vi "PRIVATE.panel.vi"() -> ()   [LabVIEW 2014]
doc: "example GUI for a class inherited from the DeviceBaseGUI\n\nauthor: Dietrich Beck, GSI\nlicense: GPL"
uses:
  CSCore/CSSystem/CoreLib/CoreLib.lvlib
  CSCore/CSObj/CSObj.lvlib
  CSlibraries/UtilityLib/UtilityLib.lvlib
  CSCore/CSApplicationBaseClasses/DeviceBase/DeviceBase.lvlib
  CSCore/CSSystem/CoreLib/CoreLib.short 2 byte array.vi
  CSCore/CSSystem/CoreLib/CoreLib.string 2 byte array.vi
  CSlibraries/UtilityLib/UtilityLib.valueStatus.ctl
  lib.lib/DimLVEvent/DimIndicators/DimIndicators.numericType.ctl
  lib.lib/DimLVEvent/DimIndicators/DimIndicators.anyType.ctl
panel:
  in  "Set":bool
  out "Busy":bool
  out "ErrorString":string
  out "deviceIDString":string
  in  "tab":enum32{"standard", "advanced"}(tab)
  in  "function":u16(ring) items=["choose function", "Initialize", "Close", "Configure", "Reset", "IDQuery"]
  in  "advancedGUI":bool
  out "loop counter":i32
  out "error out":errorcluster
  in  "error in (no error)":errorcluster
  in  "object ref":refnum<vi>
  in  "state":T1 caption="dic_service_numeric"
  in  "deviceID":T2 caption="dic_service_anyType"
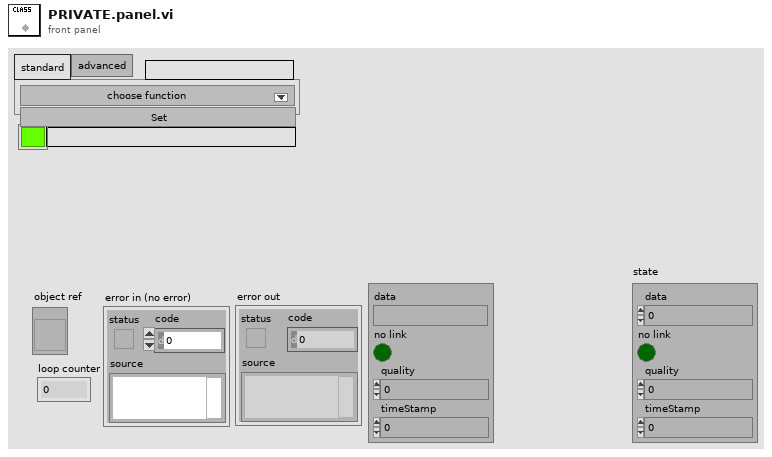
[diagram p1: front panel]
types:
  T1 = typedef "DimIndicators.lvlib/DimIndicators.numericType.ctl" = cluster{"data":dbl, "no link":bool, "quality":i32, "timeStamp":dbl}
  T2 = typedef "DimIndicators.lvlib/DimIndicators.anyType.ctl" = cluster{"data":string, "no link":bool, "quality":i32, "timeStamp":dbl}
  T3 = typedef "UtilityLib.lvlib/UtilityLib.valueStatus.ctl" = enum16{"no info available", "stand by/off", "on", "warning", "alarm/malfunction", "not implemented", "user action required", "important information", "system default", "control default", "indicator default", "button default"}
  T4 = typedef "DeviceBaseGUI.lvlib/DeviceBaseGUI.i attribute.ctl" = cluster{"GOGFrontPanel.i attribute":T5}
  T5 = typedef "GOGFrontPanel.lvlib/GOGFrontPanel.i attribute.ctl" = cluster{"GOGObject":string, "Object":string, "Method":string, "Descriptor":T6, "Input Descriptor":string, "Output Descriptor":string, "inputNames":string[], "outputNames":string[], "Values":cluster{"descriptor":string, "value":string}[]}
  T6 = typedef "BaseProcess.lvlib/BaseProcess.descriptor string definition.ctl" = string
  T7 = typedef "CoreDefs.rawDataType.ctl" = i8[]
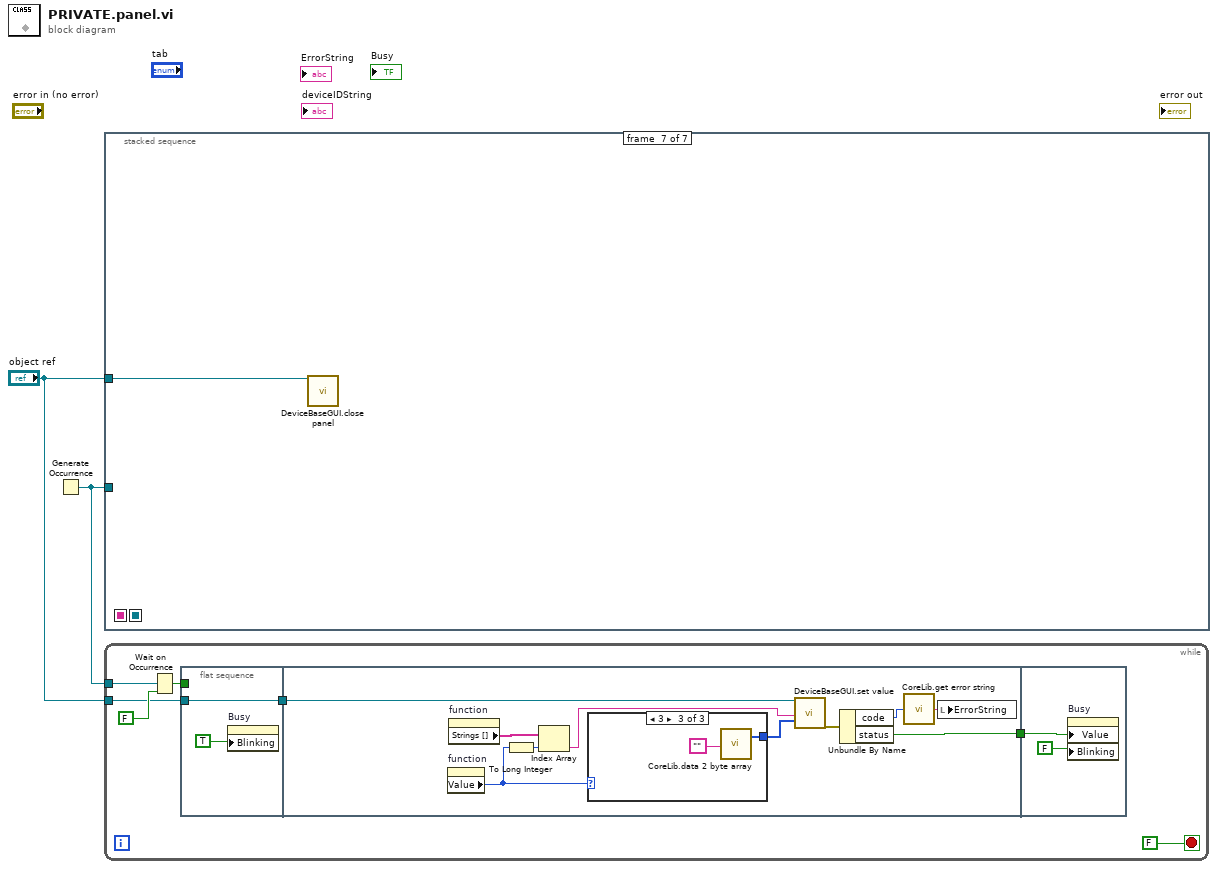
[diagram p0: block diagram]
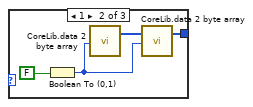
[diagram p3: hidden frame]
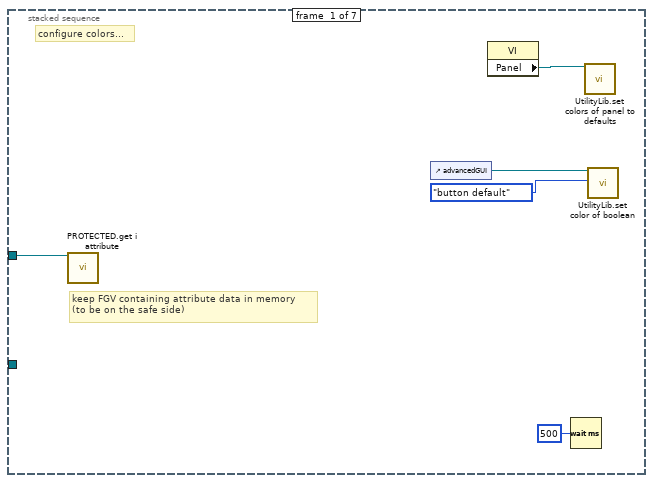
[diagram p4: hidden frame]
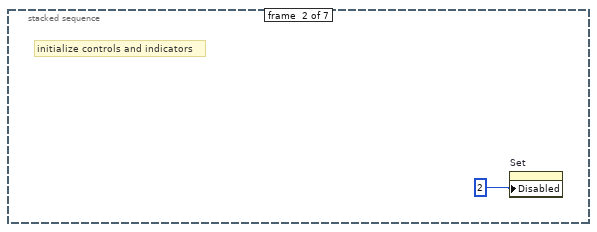
[diagram p5: hidden frame]
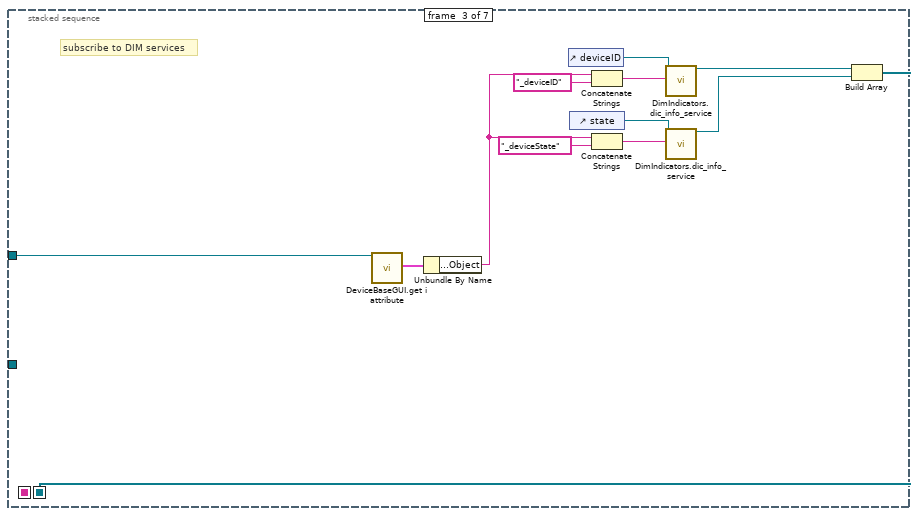
[diagram p6: hidden frame]
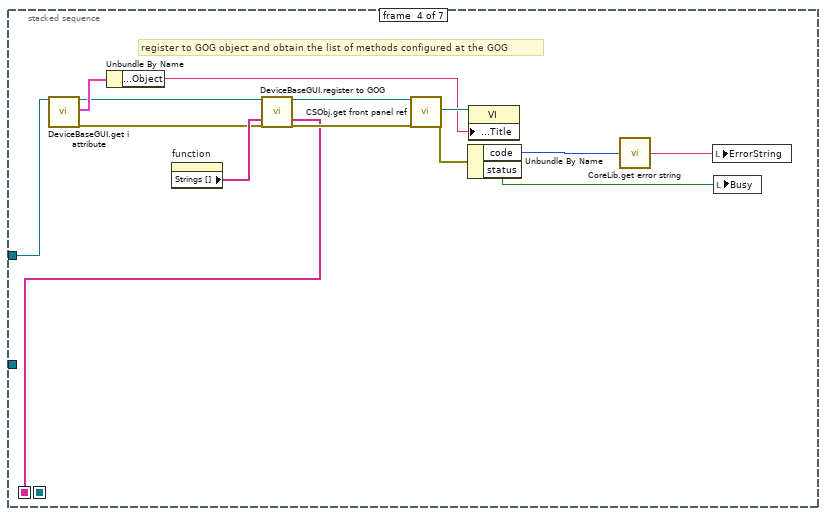
[diagram p7: hidden frame]
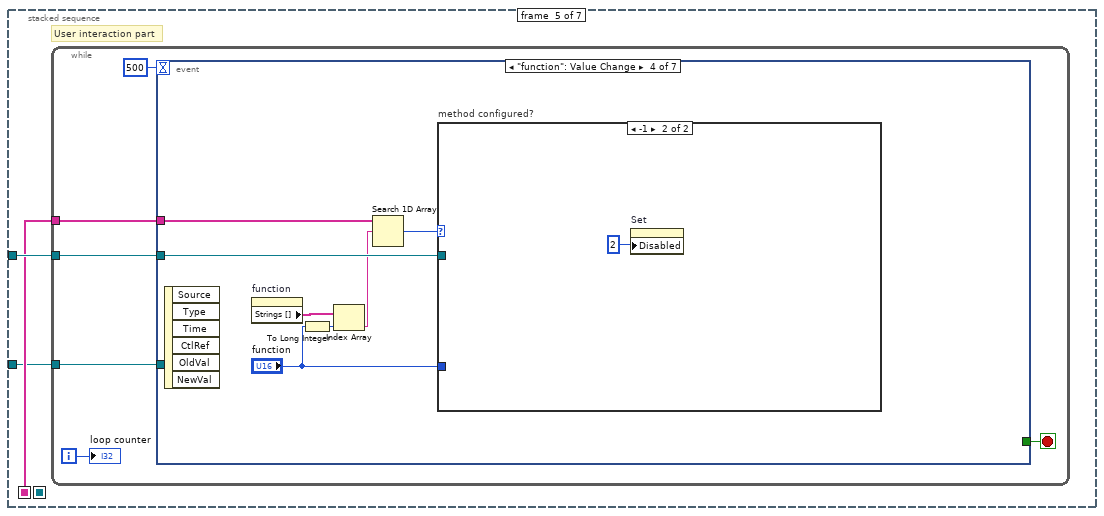
[diagram p8: hidden frame]
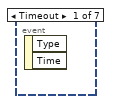
[diagram p9: hidden frame]
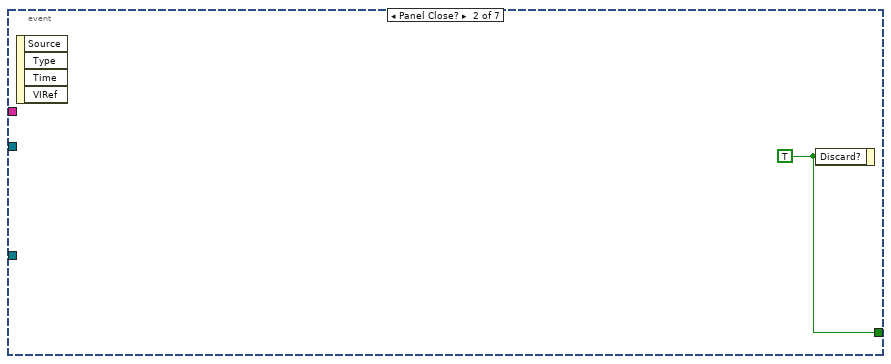
[diagram p10: hidden frame]
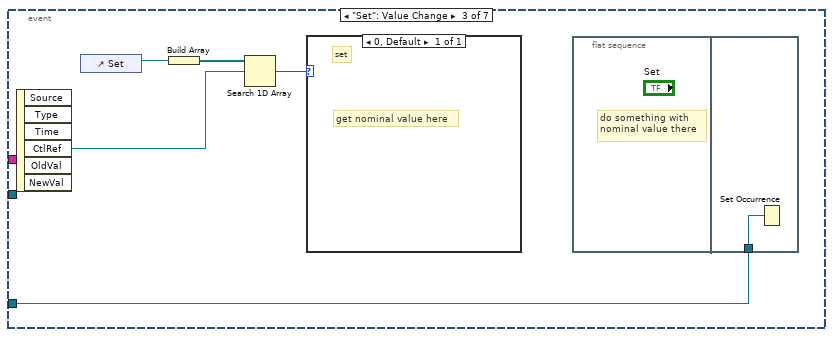
[diagram p11: hidden frame]
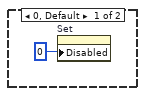
[diagram p12: hidden frame]
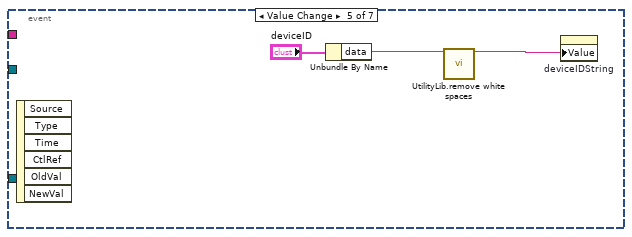
[diagram p13: hidden frame]
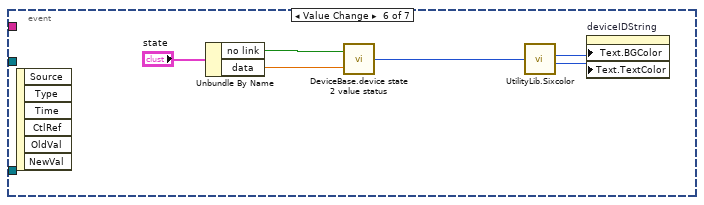
[diagram p14: hidden frame]
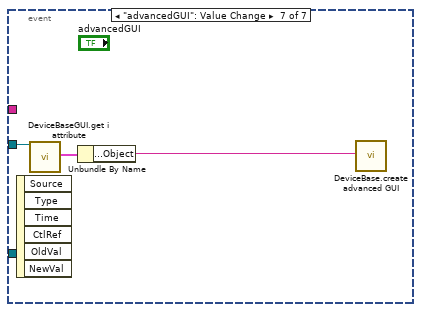
[diagram p15: hidden frame]
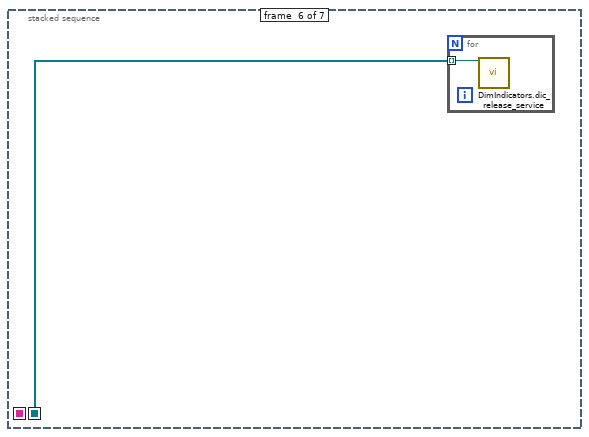
[diagram p16: hidden frame]
diagram:
  n1 = Generate Occurrence() -> (w1:refnum<k4>)
  n2 = stacked-sequence {
    seq-local: [_ _ _ w25 _ _ _] -> [_ _ _ _ w36 _ _]
    seq-local: [_ _ w9 _ _ _ _] -> [_ _ _ _ _ w72 _]
    tunnel: "object ref" -> [w3 _ w20 w34 w37 _ w74]
    tunnel: w1 -> [_ _ _ _ w35 _ _]
    frame #0 {
      # "keep FGV containing attribute data in memory\n(to be on the safe side)"
      # "configure colors..."
      n3 = call "PROTECTED.get i attribute.vi"("i ref in"=w3) -> ()  [unwired: 16 in, 3 out]
      n4 = control-ref of="advancedGUI"() -> (w5:refnum<vi>)
      n5 = property class="VI"() -> ("Panel"=w6:refnum<vi>)  [unwired: 2 in, 2 out]
      n6 = Wait (ms)(milliseconds to wait=u32 500) -> ()  [unwired: 1 out]
      n7 = call "UtilityLib.set colors of panel to defaults.vi"("Front Panel"=w6) -> ()  [unwired: 18 in, 1 out]
      n8 = call "UtilityLib.set color of boolean.vi"("button"=w5, "valueStatus"=UtilityLib.valueStatus."button default") -> ()  [unwired: 17 in, 1 out]
    }
    frame #1 {
      # "initialize controls and indicators"
      n9 = property on="Set" class="Bool"("Disabled"=u8 2) -> ()  [unwired: 2 in, 2 out]
    }
    frame #2 {
      # "subscribe to DIM services"
      n10 = call "DeviceBaseGUI.get i attribute.vi"("i ref in"=w20) -> ("i attribute"=w19:T4)  [unwired: 16 in, 2 out]
      n11 = Unbundle By Name(w19) -> ("GOGFrontPanel.i attribute.Object"=w16:string)
      n12 = control-ref of="deviceID"() -> (w14:refnum<vi>)
      n13 = control-ref of="state"() -> (w12:refnum<vi>)
      n14 = Concatenate Strings(w16, "_deviceID" ("string")) -> (w15:string)
      n15 = Concatenate Strings(w16, "_deviceState" ("string")) -> (w13:string)
      n16 = call "DimIndicators.dic_info_service.vi"("controlRef"=w14, "serviceName"=w15) -> ("controlRef out"=w11:refnum<vi>)  [unwired: 16 in, 1 out]
      n17 = call "DimIndicators.dic_info_service.vi"("controlRef"=w12, "serviceName"=w13) -> ("controlRef out"=w10:refnum<vi>)  [unwired: 16 in, 1 out]
      n18 = Build Array(w11, w10) -> (w9:refnum<vi>[])
    }
    frame #3 {
      # "register to GOG object and obtain the list of methods configured at the GOG"
      n19 = call "DeviceBaseGUI.get i attribute.vi"("i ref in"=w34) -> ("i ref out"=w30:refnum<vi>, "i attribute"=w33:T4, "error out"=w27:errorcluster)  [unwired: 16 in]
      n20 = Unbundle By Name(w33) -> ("GOGFrontPanel.i attribute.Object"=w31:string)
      n21 = property on="function" class="Ring (strict)"() -> ("Strings []"=w28:string[])  [unwired: 2 in, 2 out]
      n22 = call "DeviceBaseGUI.register to GOG.vi"("i ref in"=w30, "myMethods"=w28, "error in (no error)"=w27) -> ("i ref out"=w29:refnum<vi>, "configuredMethods"=w25:string[], "error out"=w26:errorcluster)  [unwired: 14 in]
      n23 = call "CSObj.get front panel ref.vi"("i ref in"=w29, "error in (no error)"=w26) -> ("frontPanelRef"=w32:refnum<vi>, "error out"=w21:errorcluster)  [unwired: 15 in, 1 out]
      n24 = Unbundle By Name(w21) -> ("code"=w24:i32, "status"=w22:bool)
      n25 = property class="VI"(reference=w32, "Front Panel Window:Title"=w31) -> ()  [unwired: 1 in, 2 out]
      n26 = call "CoreLib.get error string.vi"("Error Code"=w24) -> ("Error String"=w23:string)
      n27 = local write "ErrorString"(w23) -> ()
      n28 = local write "Busy"(w22) -> ()
    }
    frame #4 {
      # "User interaction part"
      n29 = while {
        tunnel: w37 -> [w42]
        tunnel: w36 -> [w40]
        tunnel: w35 -> [w39]
        i -> [w43]
        stop <- w38 stop-if-true
        n30 = event shown="[3] \"function\": Value Change" {
          selector: _ -> [_ _ _ _ _ _ _]
          dyn-events: _ -> [_ _ _ _ _ _ _]
          timeout: 500 -> [_ _ _ _ _ _ _]
          tunnel: w42 -> [_ _ _ w57 _ _ w70]
          tunnel: w40 -> [_ _ _ w55 _ _ _]
          tunnel: w39 -> [_ _ w45 _ _ _ _]
          tunnel: [_ w44 _ _ _ _ _] -> w38
          event Timeout {
            n31 = event-data() -> ()  [unwired: 1 in, 2 out]
          }
          event Panel Close? {
            w44 = TRUE ("Discard?")
            n32 = event-data() -> ()  [unwired: 1 in, 4 out]
            n33 = event-data("Discard?"=w44) -> ()  [unwired: 1 in, 1 out]
          }
          event "Set": Value Change {
            n34 = event-data() -> ("CtlRef"=w47:refnum<vi>)  [unwired: 1 in, 5 out]
            n35 = control-ref of="Set"() -> (w49:refnum<vi>)
            n36 = Build Array(w49) -> (w48:refnum<vi>[])
            n37 = Search 1D Array(1D array=w48, element=w47) -> (index of element=w46:i32)  [unwired: 1 in]
            n38 = case shown="0, Default" w46 {
              frame 0, Default {
                # "get nominal value here"
                # "set"
              }
            }
            n39 = flat-sequence {
              tunnel: w45 -> [w50]
              frame #0 {
                # "do something with\nnominal value there"
              }
              frame #1 {
                n40 = Set Occurrence(w50) -> ()
              }
            }
          }
          event "function": Value Change {
            n41 = event-data() -> ()  [unwired: 1 in, 6 out]
            n42 = property on="function" class="Ring (strict)"() -> ("Strings []"=w56:string[])  [unwired: 2 in, 2 out]
            n43 = To Long Integer(number="function") -> (32bit integer=w51:i32)
            n44 = Index Array(array=w56, index=w51) -> (element=w54:string)
            n45 = Search 1D Array(1D array=w55, element=w54) -> (index of element=w53:i32)  [unwired: 1 in]
            n46 = case "method configured?" shown="-1" w53 {
              tunnel: w57 -> [_ _]
              tunnel: "function" -> [_ _]
              frame 0, Default {
                n47 = property on="Set" class="Bool"("Disabled"=u8 0) -> ()  [unwired: 2 in, 2 out]
              }
              frame -1 {
                n48 = property on="Set" class="Bool"("Disabled"=u8 2) -> ()  [unwired: 2 in, 2 out]
              }
            }
          }
          event Value Change {
            n49 = event-data() -> ()  [unwired: 1 in, 6 out]
            n50 = Unbundle By Name("deviceID") -> ("data"=w62:string)
            n51 = call "UtilityLib.remove white spaces.vi"("string with blanks"=w62) -> ("string without white spaces"=w61:string)  [unwired: 14 in, 4 out]
            n52 = property on="deviceIDString" class="Str"("Value"=w61) -> ()  [unwired: 2 in, 2 out]
          }
          event Value Change {
            n53 = event-data() -> ()  [unwired: 1 in, 6 out]
            n54 = Unbundle By Name("state") -> ("no link"=w68:bool, "data"=w65:dbl)
            n55 = call "DeviceBase.device state 2 value status.vi"("deviceState"=w65, "no link"=w68) -> ("valueStatus"=w67:T3)
            n56 = call "UtilityLib.Sixcolor.vi"("State"=w67) -> ("elementBackground"=w66:u32, "elementText"=w63:u32)  [unwired: 2 in, 2 out]
            n57 = property on="deviceIDString" class="Str"("Text.BGColor"=w66, "Text.TextColor"=w63) -> ()  [unwired: 2 in, 2 out]
          }
          event "advancedGUI": Value Change {
            n58 = event-data() -> ()  [unwired: 1 in, 6 out]
            n59 = call "DeviceBaseGUI.get i attribute.vi"("i ref in"=w70) -> ("i attribute"=w71:T4)  [unwired: 16 in, 2 out]
            n60 = Unbundle By Name(w71) -> ("GOGFrontPanel.i attribute.Object"=w69:string)
            n61 = call "DeviceBase.create advanced GUI.vi"("Object"=w69) -> ()  [unwired: 17 in, 2 out]
          }
        }
        "loop counter" <- w43
      }
    }
    frame #5 {
      n62 = for {
        tunnel: w72 -> [w73] mode=indexing
        n63 = call "DimIndicators.dic_release_service.vi"("controlRef"=w73) -> ()  [unwired: 18 in, 1 out]
      }
    }
    frame #6 {
      n64 = call "DeviceBaseGUI.close panel.vi"("i ref in"=w74) -> ()  [unwired: 17 in, 2 out]
    }
  }
  n65 = while {
    tunnel: w1 -> [w79]
    tunnel: "object ref" -> [w76]
    stop <- FALSE stop-if-true
    n66 = Wait on Occurrence(1:FALSE ("ignore previous (T)"), 2:w79) -> (0:w78:bool)  [unwired: 1 in]
    n67 = flat-sequence {
      tunnel: w78 -> [_]
      tunnel: [w82] -> w77
      tunnel: w76 -> [w82]
      tunnel: w77 -> [w87]
      tunnel: [w86] -> w75
      tunnel: w75 -> [w100]
      frame #0 {
        n68 = property on="Busy" class="Bool (strict)"("Blinking"=TRUE) -> ()  [unwired: 2 in, 2 out]
      }
      frame #1 {
        n69 = property on="function" class="Ring (strict)"() -> ("Value"=w93:u16)  [unwired: 2 in, 2 out]
        n70 = property on="function" class="Ring (strict)"() -> ("Strings []"=w91:string[])  [unwired: 2 in, 2 out]
        n71 = To Long Integer(number=w93) -> (32bit integer=w85:i32)
        n72 = Index Array(array=w91, index=w85) -> (element=w84:string)
        n73 = case shown="3" w93 {
          tunnel: [_ w97 w99] -> w92
          frame 0, Default {
          }
          frame 1 {
            n74 = Boolean To (0,1)(Boolean=FALSE) -> (0, 1=w95:i16)
            n75 = call-poly "CoreLib.data 2 byte array.vi"("i16"=w95) -> ("byteArray out"=w96:T7)  [unwired: 18 in]
            n76 = call-poly "CoreLib.data 2 byte array.vi"("byteArray"=w96, "i16"=w95) -> ("byteArray out"=w97:T7)  [unwired: 17 in]
          }
          frame 3 {
            n77 = call-poly "CoreLib.data 2 byte array.vi"("string"="") -> ("byteArray out"=w99:T7)  [unwired: 18 in]
          }
        }
        n78 = call "DeviceBaseGUI.set value.vi"("i ref in"=w87, "methodName"=w84, "byteArray"=w92) -> ("error out"=w89:errorcluster)  [unwired: 15 in, 1 out]
        n79 = Unbundle By Name(w89) -> ("code"=w90:i32, "status"=w86:bool)
        n80 = call "CoreLib.get error string.vi"("Error Code"=w90) -> ("Error String"=w88:string)
        n81 = local write "ErrorString"(w88) -> ()
      }
      frame #2 {
        n82 = property on="Busy" class="Bool (strict)"("Value"=w100, "Blinking"=FALSE) -> ()  [unwired: 2 in, 2 out]
      }
    }
  }
